vi "GetLimsTestSteps.vi"(8 "error in (no error)":errorcluster, 10 "test-id":i32, 11 "ByteGSAPIBase in":refnum<class "ByteGSAPIBase.lvclass">) -> (0 "error out":errorcluster, 2 "list of steps":T1[](array[typedef]), 3 "ByteGSAPIBase out":refnum<class "ByteGSAPIBase.lvclass">)   [LabVIEW 2019, in "ByteGSWebAPI.lvlib" / "ByteGSAPIBase.lvclass"]
doc: "Obtain the list of steps for a Test based on the test-id"
uses:
  ByteGSAPIBase.lvclass
  TypeDef/Step.ctl
  TypeDef/Asset.ctl
  ByteGSAPIBase.lvclass/ByteGSAPIBase.ctl
  <vilib>/Bytelabs/ByteREST/ByteRESTClass/ByteRESTBase/RESTBase.lvclass
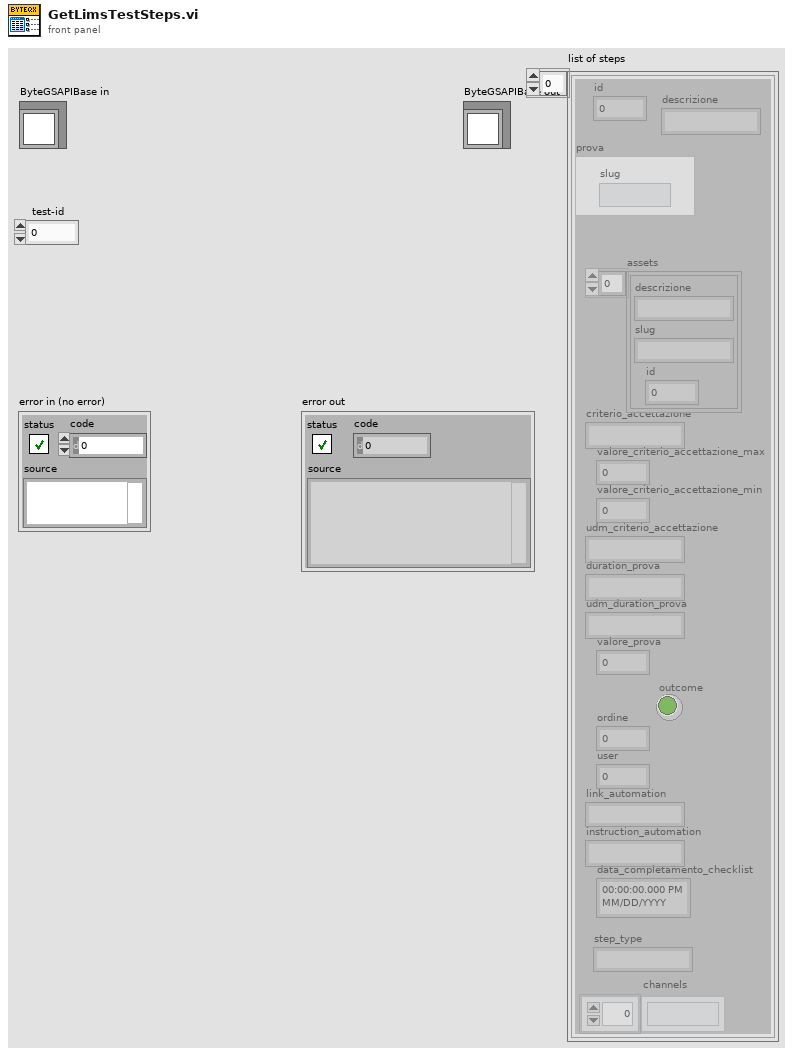
[diagram p1: front panel]
types:
  T1 = typedef "ByteGSWebAPI.lvlib/ByteGSAPIBase.lvclass/Step.ctl" = cluster{"id":i32, "descrizione":string, "prova":cluster{"slug":string}, "assets":T2[], "criterio_accettazione":string, "valore_criterio_accettazione_max":dbl, "valore_criterio_accettazione_min":dbl, "udm_criterio_accettazione":string, "duration_prova":string, "udm_duration_prova":string, "valore_prova":dbl, "ordine":i32, "user":i32, "link_automation":string, "instruction_automation":string, "data_completamento_checklist":timestamp, "outcome":bool, "step_type":string, "channels":string[]}
  T2 = typedef "ByteGSWebAPI.lvlib/ByteGSAPIBase.lvclass/Asset.ctl" = cluster{"descrizione":string, "slug":string, "id":i32}
  T3 = cluster{"id":i32, "descrizione":string, "prova":cluster{"slug":string}, "assets":T2[], "criterio_accettazione":string, "valore_criterio_accettazione_max":dbl, "valore_criterio_accettazione_min":dbl, "udm_criterio_accettazione":string, "duration_prova":string, "udm_duration_prova":string, "data_completamento_checklist":string, "valore_prova":dbl, "outcome":string, "ordine":i32, "user":i32, "link_automation":string, "instruction_automation":string}[]
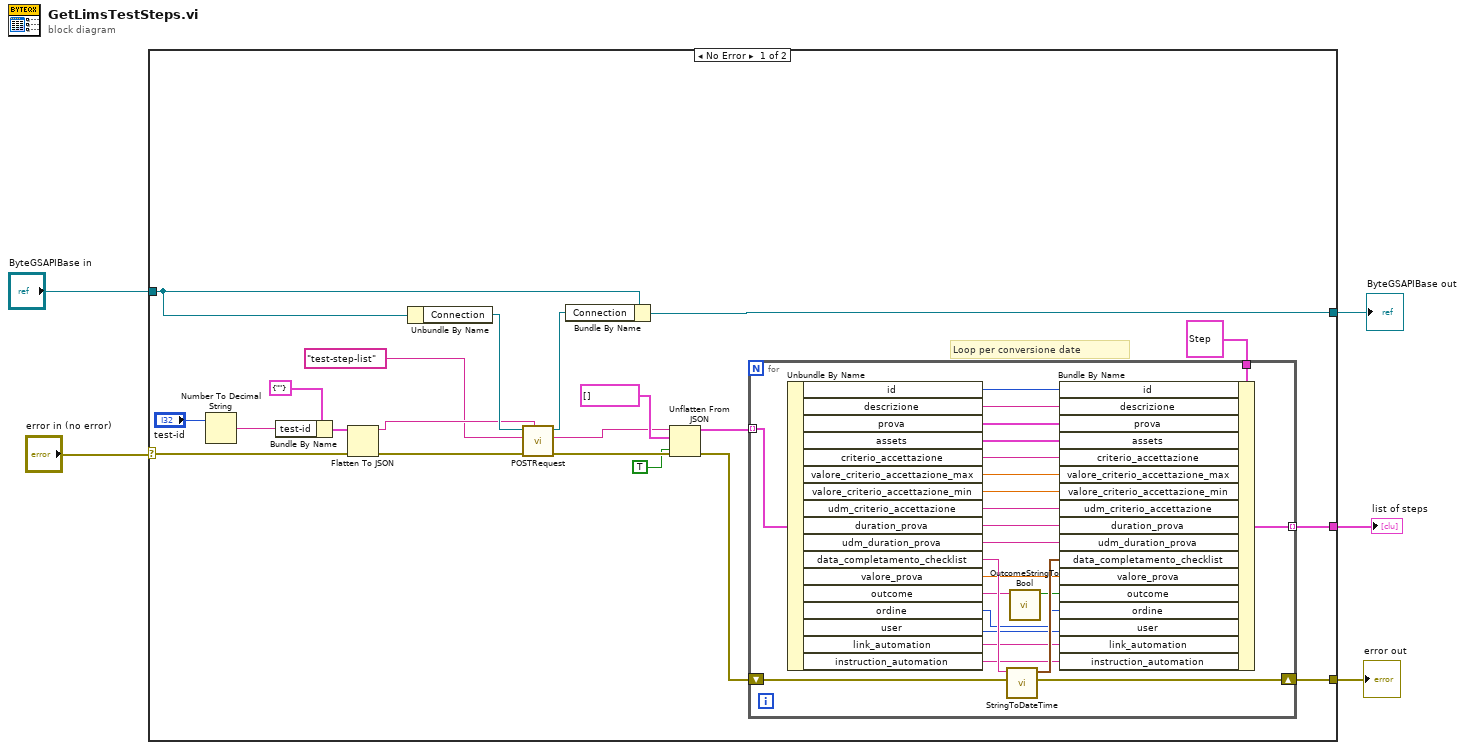
[diagram p0: block diagram]
diagram:
  n1 = case shown="No Error" "error in (no error)" {
    selector: "error in (no error)" -> [w23 w52]
    tunnel: [w8 w52] -> w4
    tunnel: [w24 w51] -> w2
    tunnel: "ByteGSAPIBase in" -> [w15 w51]
    tunnel: [w6 _] -> w1
    frame No Error {
      # "Loop per conversione date"
      n2 = Number To Decimal String(number="test-id") -> (decimal integer string=w13:string)  [unwired: 1 in]
      n3 = Bundle By Name(cluster=cluster{"test-id":string} {"test-id"=""} ("Request"), "test-id"=w13) -> (w12:cluster{"test-id":string})
      n4 = Flatten To JSON(anything=w12, error in (no error)=w23) -> (JSON string=w21:string, 11:w25:errorcluster)  [unwired: 1 in]
      n5 = Unbundle By Name(w15) -> ("Connection"=w26:refnum<class "RESTBase.lvclass">)
      n6 = call-dynamic "POSTRequest.vi"("Body in"=w21, "error in (no error)"=w25, "Request"="test-step-list", "ByteRESTBase in"=w26) -> ("error out"=w19:errorcluster, "Body"=w17:string, "ByteRESTBase out"=w18:refnum<class "RESTBase.lvclass">)  [unwired: 4 in, 1 out]
      n7 = Bundle By Name(cluster=w15, "Connection"=w18) -> (w24:refnum<class "ByteGSAPIBase.lvclass">)
      n8 = Unflatten From JSON(JSON string=w17, type and defaults=T3 [], default null elements? (F)=TRUE, error in (no error)=w19) -> (value=w11:T3, error out=w9:errorcluster)  [unwired: 3 in]
      n9 = for {
        tunnel: w11 -> [w50] mode=indexing
        tunnel: T1 {"id"=0, "descrizione"="", "prova"={"slug"=""}, "assets"=[], "criterio_accettazione"="", "valore_criterio_accettazione_max"=0.0, "valore_criterio_accettazione_min"=0.0, "udm_criterio_accettazione"="", "duration_prova"="", "udm_duration_prova"="", "valore_prova"=0.0, "ordine"=0, "user"=0, "link_automation"="", "instruction_automation"="", "data_completamento_checklist"=timestamp(0 s since 1904-01-01), "outcome"=FALSE, "step_type"="", "channels"=[]} -> [w49]
        shift-right: [w30] -> w8
        shift-left: w9 -> [w31]
        tunnel: [w29] -> w6 mode=indexing
        n10 = Unbundle By Name(w50) -> ("id"=w48:i32, "descrizione"=w47:string, "prova"=w46:cluster{"slug":string}, "assets"=w45:T2[], "criterio_accettazione"=w44:string, "valore_criterio_accettazione_max"=w43:dbl, "valore_criterio_accettazione_min"=w42:dbl, "udm_criterio_accettazione"=w41:string, "duration_prova"=w40:string, "udm_duration_prova"=w39:string, "data_completamento_checklist"=w38:string, "valore_prova"=w36:dbl, "outcome"=w28:string, "ordine"=w35:i32, "user"=w34:i32, "link_automation"=w33:string, "instruction_automation"=w32:string)
        n11 = call "StringToDateTime.vi"("error in (no error)"=w31, "datetime string"=w38) -> ("error out"=w30:errorcluster, "timestamp"=w37:timestamp)  [unwired: 8 in]
        n12 = call "OutcomeStringToBool.vi"("outcome string"=w28) -> ("outcome bool"=w27:bool)  [unwired: 10 in]
        n13 = Bundle By Name(cluster=w49, "id"=w48, "descrizione"=w47, "prova"=w46, "assets"=w45, "criterio_accettazione"=w44, "valore_criterio_accettazione_max"=w43, "valore_criterio_accettazione_min"=w42, "udm_criterio_accettazione"=w41, "duration_prova"=w40, "udm_duration_prova"=w39, "data_completamento_checklist"=w37, "valore_prova"=w36, "outcome"=w27, "ordine"=w35, "user"=w34, "link_automation"=w33, "instruction_automation"=w32) -> (w29:T1)
      }
    }
    frame Error {
    }
  }
  "error out" <- w4
  "ByteGSAPIBase out" <- w2
  "list of steps" <- w1
